vi "FPGA.vi"(8 "Servo PWM":i16, 9 "Motor PWM":i16=97, 13 "Slave Address":u8 format="%x", 15 "Data to send":u8[](array[numeric])=[0, 0] format="%b", 17 "Number of bytes":i16) -> (12 "Block Count":i16, 14 "Time of Flight Right":u32, 19 "Data bit array":bool[](array[boolean]), 20 "Time of Flight Front":u32, 24 "Time of Flight Back":u32, 26 "Time of Flight Left":u32)   [LabVIEW 2015]
uses:
  <vilib>/rvi/Emulation/niFpgaGetClockAttributes.vi
  <vilib>/rvi/Emulation/niFpgaSctlEmulationGetInTimedLoop.vi
  <vilib>/rvi/Emulation/niFpgaEmulationReportErrorSimple.vi
  <vilib>/rvi/eio/common/nirviEmuTemplateMethod_errors.vi
  <vilib>/rvi/Emulation/niFpgaCriticalErrorInLSC.vi
  <vilib>/rvi/Emulation/niFpgaProcessEmulError.vi
  <vilib>/eio/EIONode/EIONode.xnode
panel:
  out "Waveform Chart 2":i16(graph)
  out "Waveform Chart":i16(graph)
  in  "Read":bool=TRUE
  out "x*y 4":i16
  out "x*y 3":i16
  out "x*y 2":i16
  out "x*y":i16
  in  "stop":bool
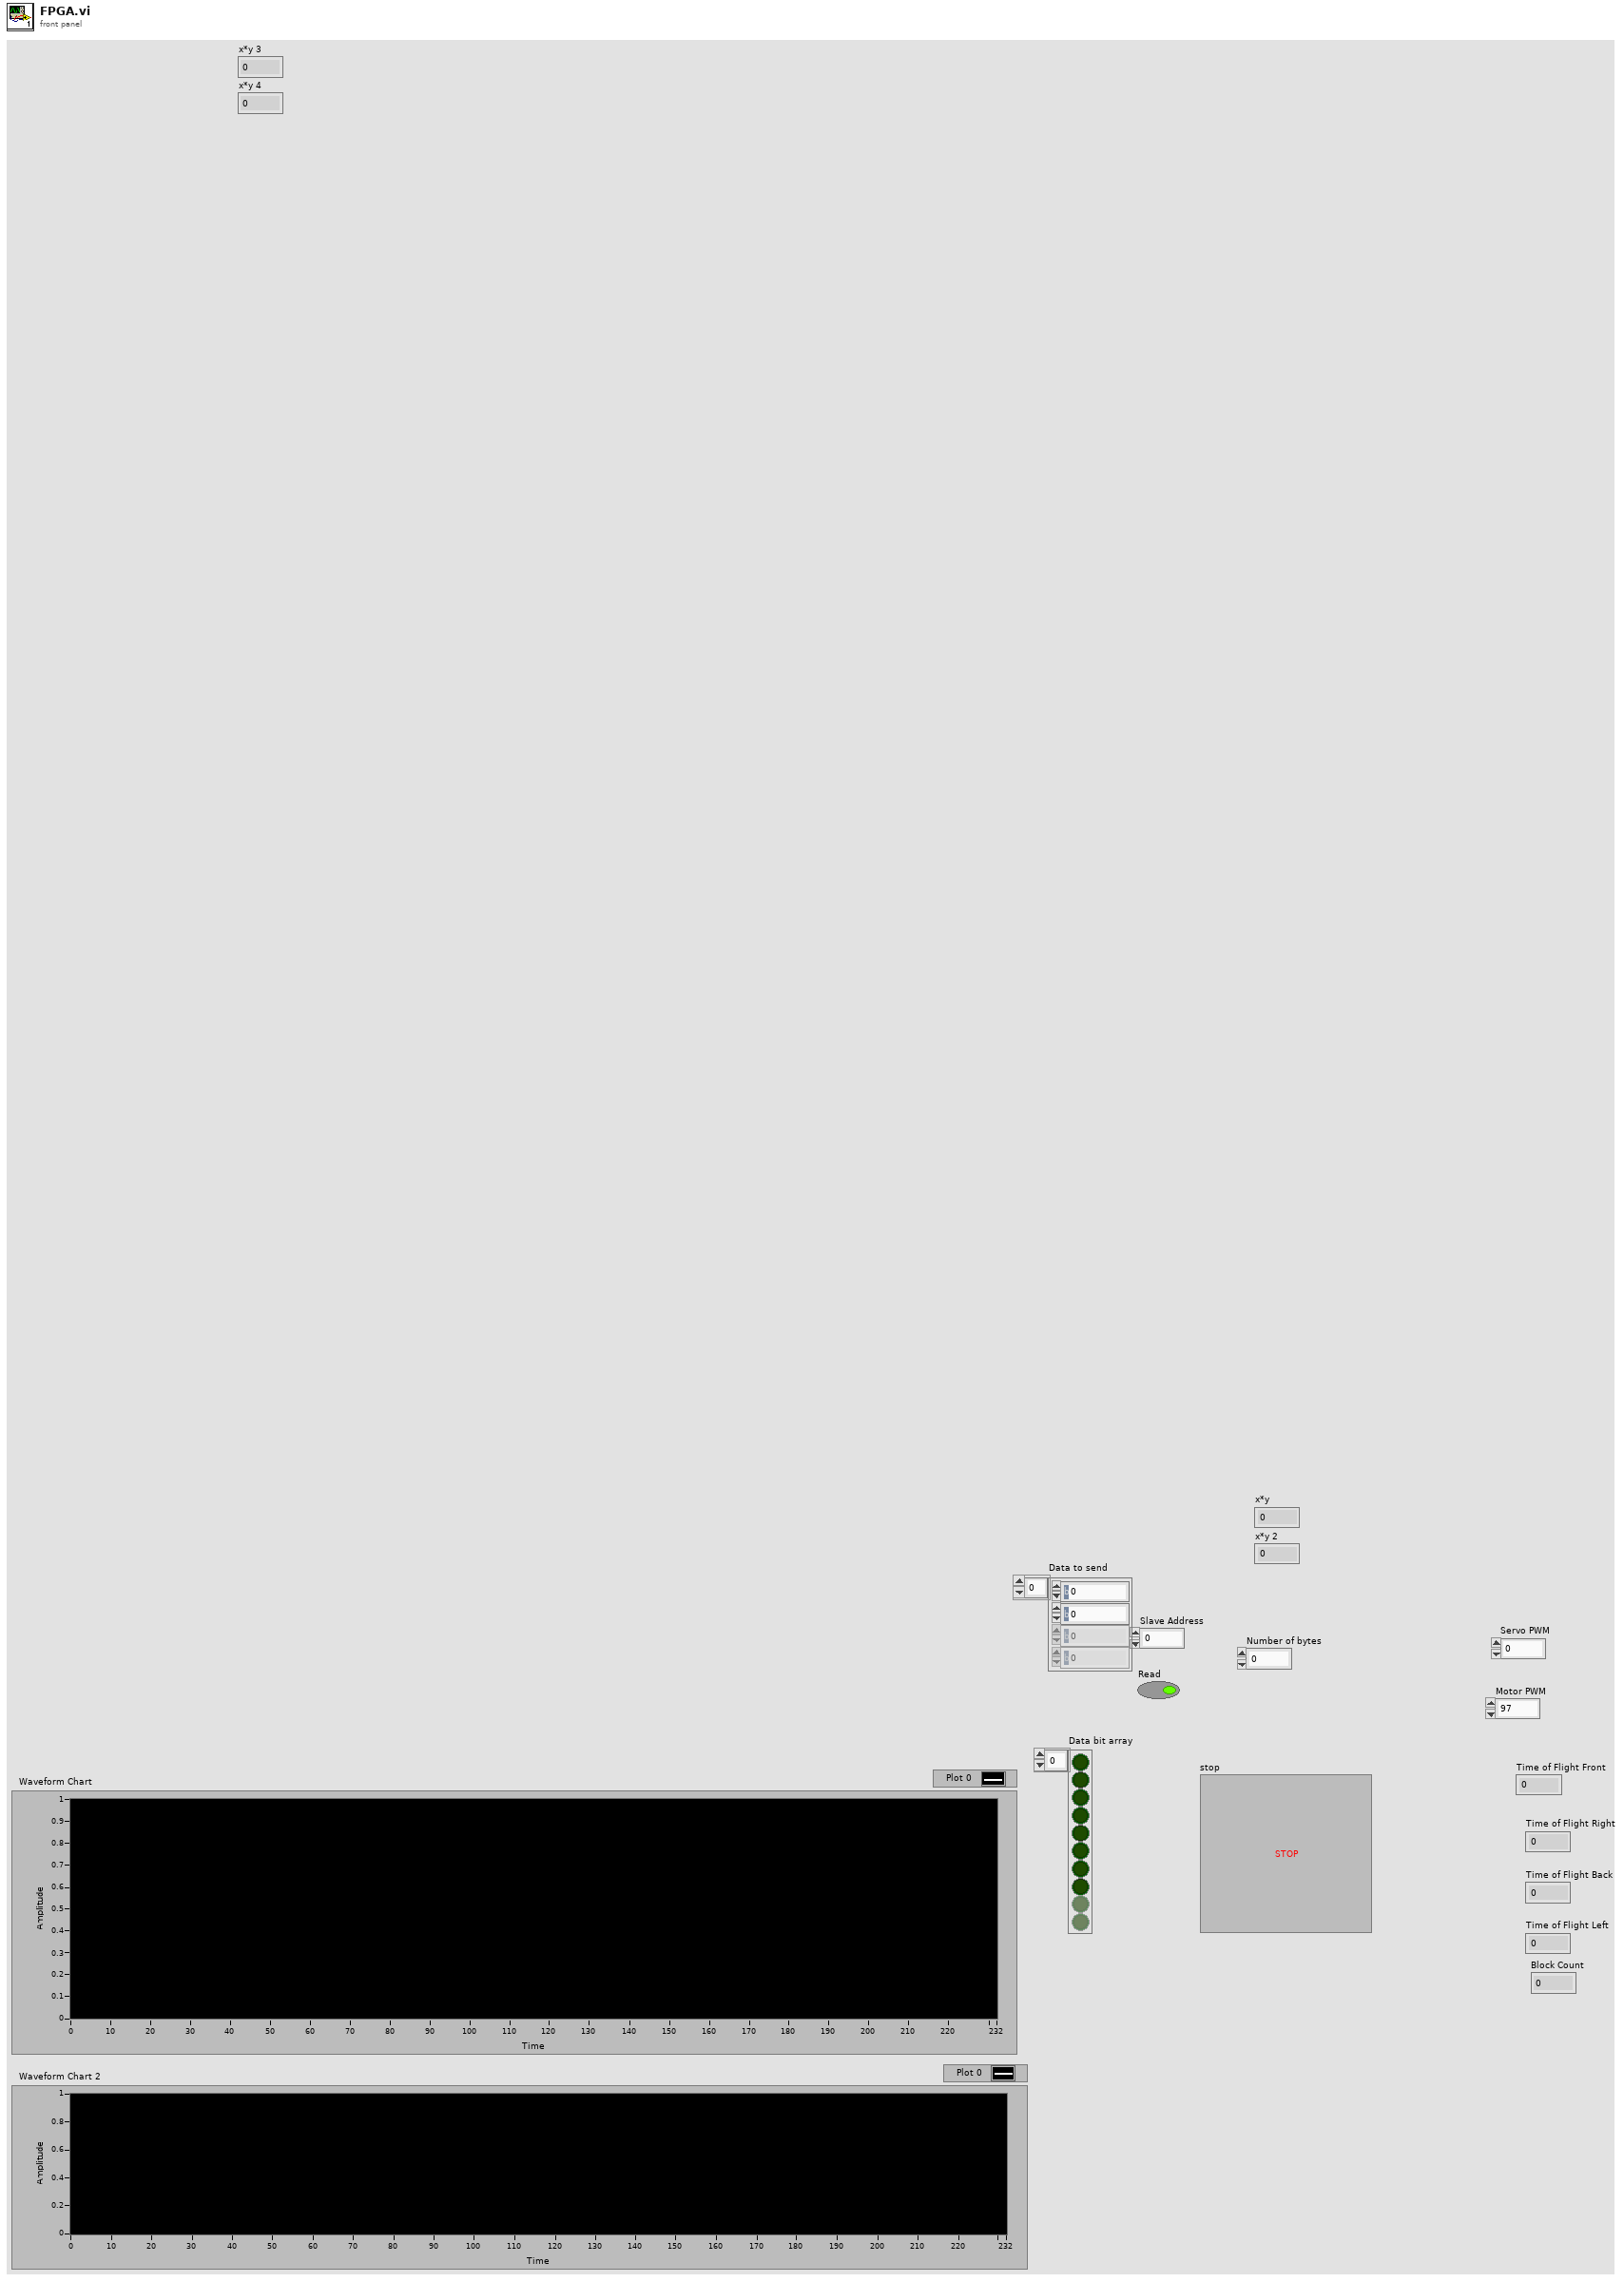
[diagram p1: front panel]
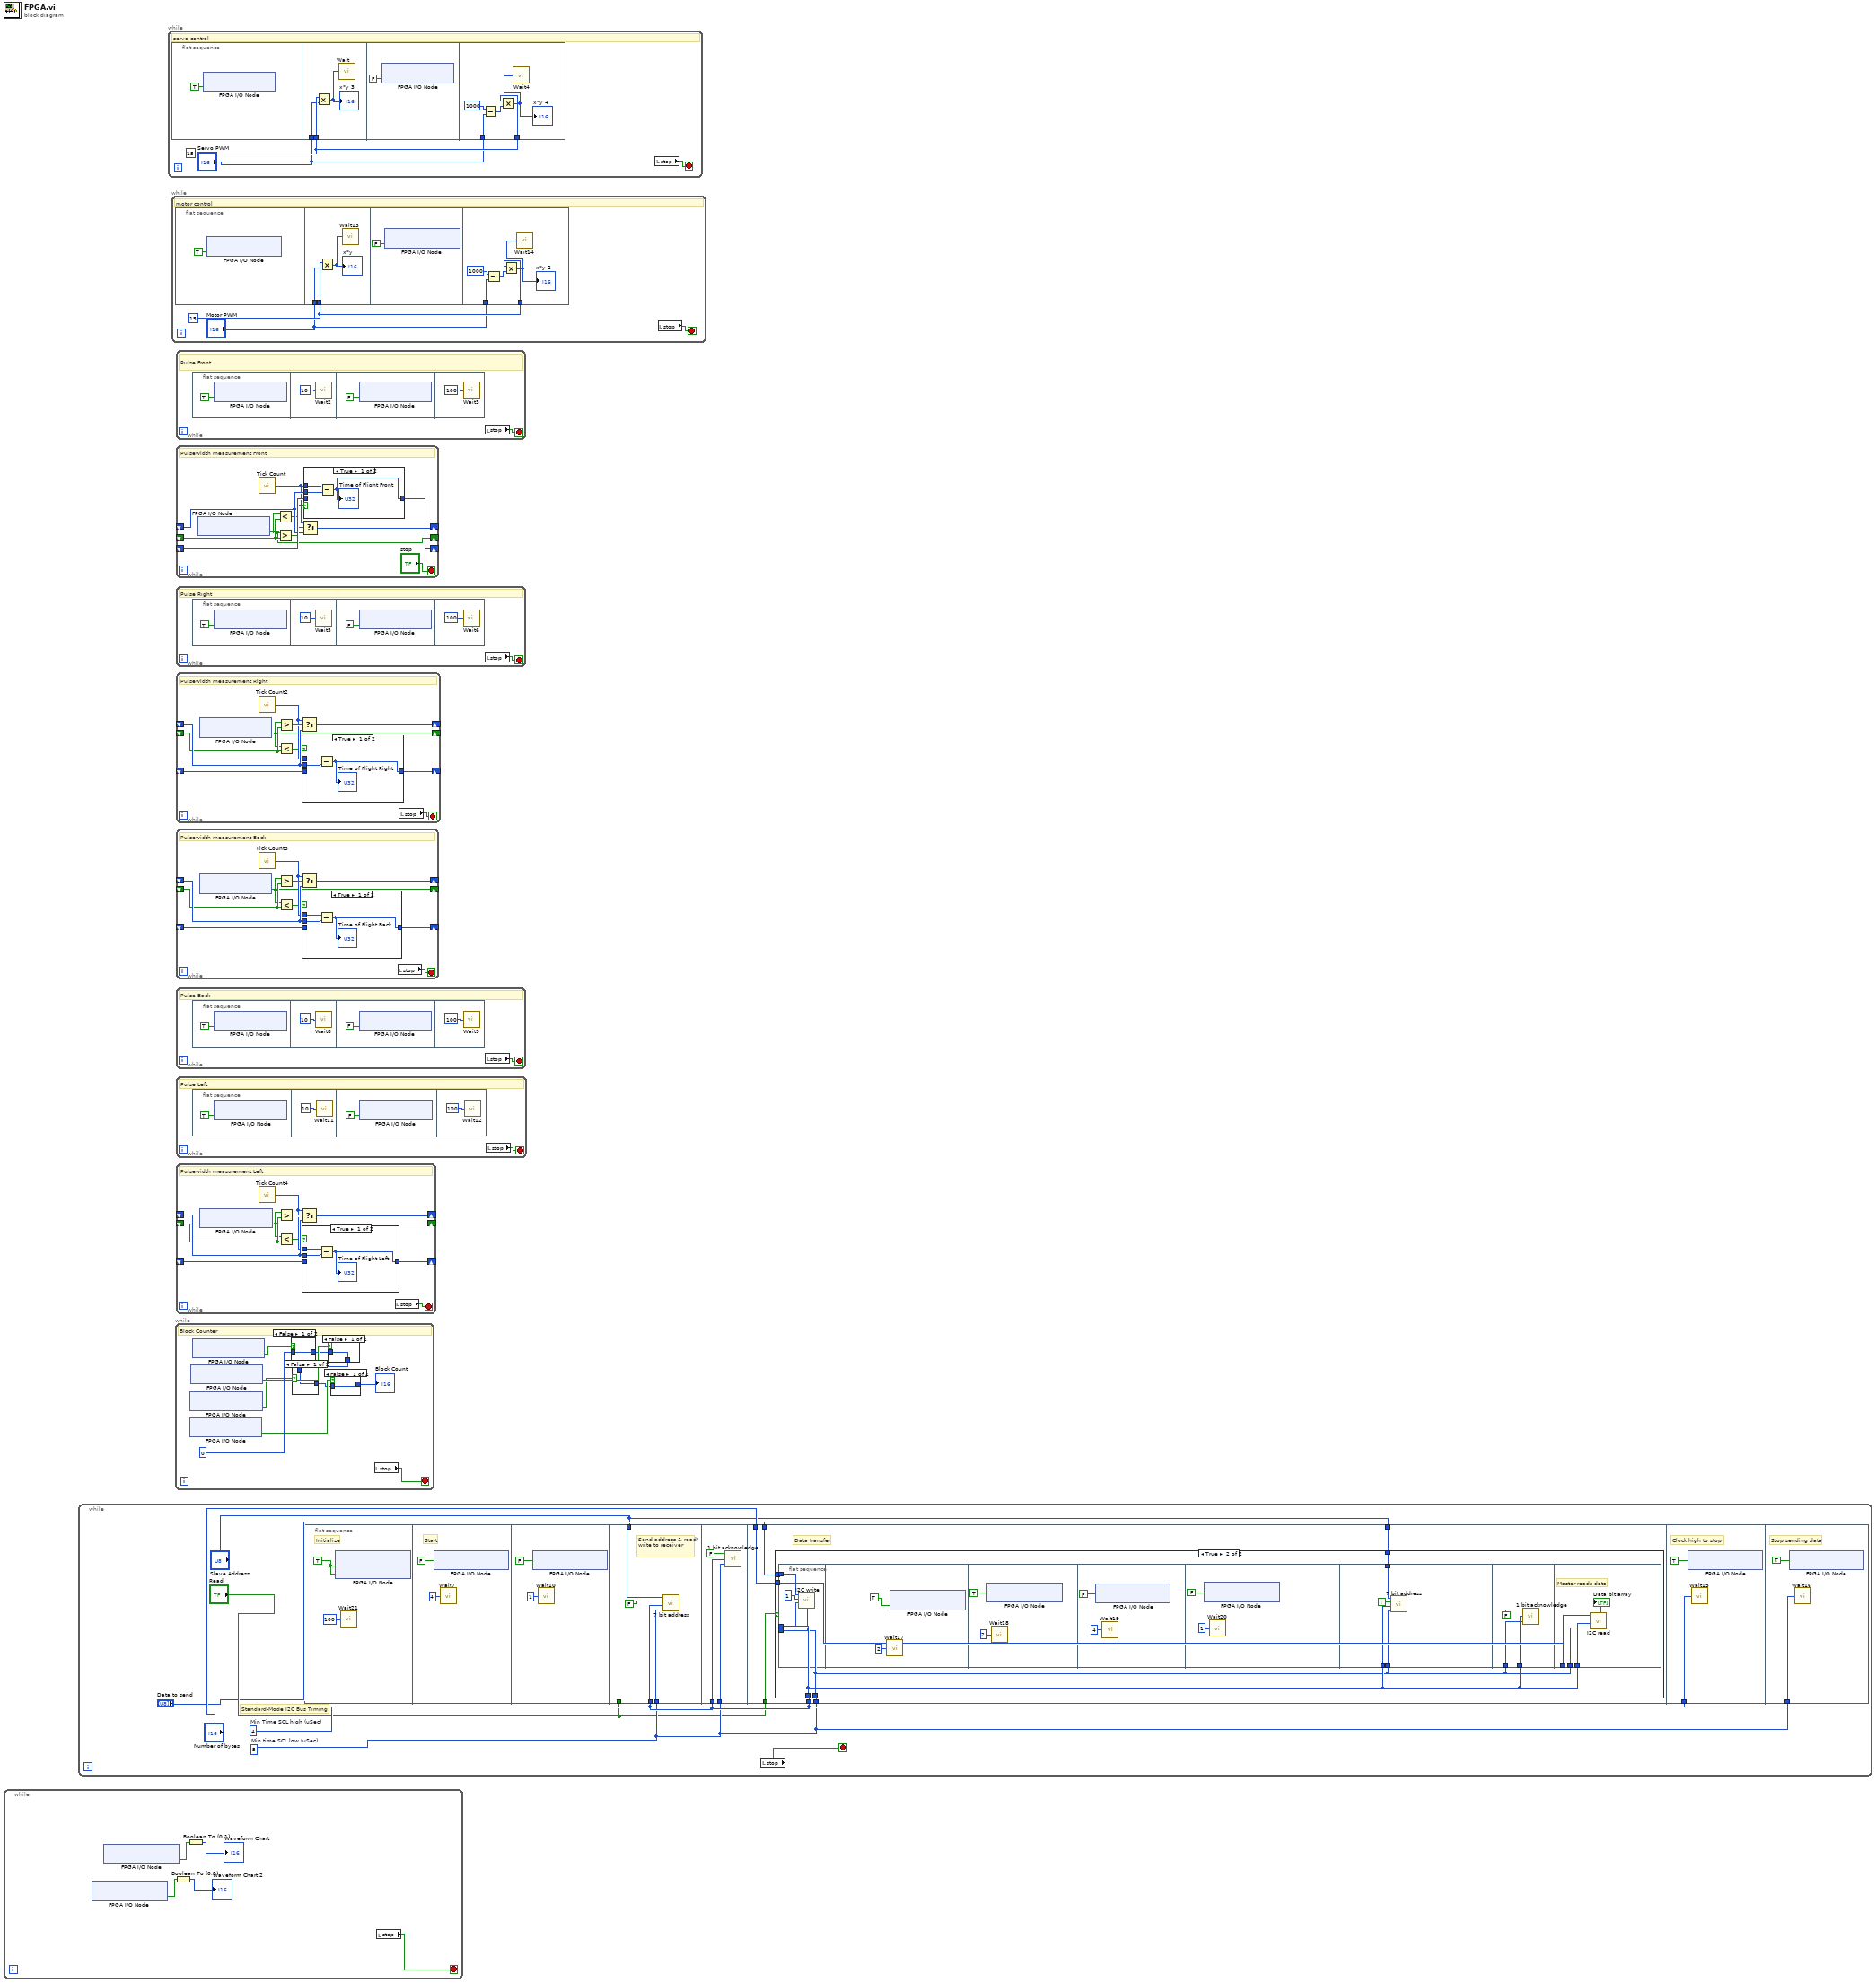
[diagram p0: block diagram]
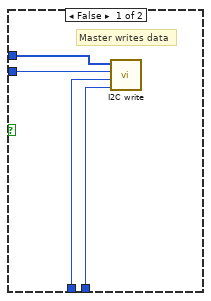
[diagram p2: hidden frame]
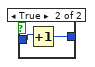
[diagram p3: hidden frame]
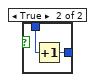
[diagram p4: hidden frame]
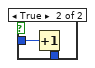
[diagram p5: hidden frame]
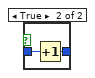
[diagram p6: hidden frame]
diagram:
  n1 = while {
    stop <- w5 stop-if-true
    n2 = xnode "FPGA I/O Node"() -> ("ConnectorB/DIO14"=w2:bool)  [unwired: 1 in, 1 out]
    n3 = xnode "FPGA I/O Node"() -> ("ConnectorB/DIO15"=w4:bool)  [unwired: 1 in, 1 out]
    n4 = Boolean To (0,1)(Boolean=w2) -> (0, 1=→"Waveform Chart 2":i16)
    n5 = Boolean To (0,1)(Boolean=w4) -> (0, 1=→"Waveform Chart":i16)
    n6 = local read "stop"() -> (w5:bool)
  }
  n7 = while {
    stop <- w12 stop-if-true
    w11 = 4  # Min Time SCL high (uSec)
    w10 = 5  # Min time SCL low (uSec)
    # "Standard-Mode I2C Bus Timing"
    n8 = flat-sequence {
      tunnel: "Read" -> [_]
      tunnel: w11 -> [w22]
      tunnel: w10 -> [w21]
      tunnel: "Slave Address" -> [w20]
      tunnel: w11 -> [w24]
      tunnel: w10 -> [w23]
      tunnel: "Read" -> [w31]
      tunnel: w11 -> [w30]
      tunnel: w10 -> [w29]
      tunnel: "Data to send" -> [w28]
      tunnel: "Number of bytes" -> [w27]
      tunnel: "Slave Address" -> [w26]
      tunnel: w11 -> [w64]
      tunnel: w10 -> [w67]
      frame #0 {
        w14 = TRUE ("Digital Out")
        # "Initialize"
        n9 = xnode "FPGA I/O Node"("ConnectorB/DIO15"=w14, "ConnectorB/DIO14"=w14) -> ()  [unwired: 2 in, 2 out]
        n10 = call "Wait21"("Count(uSec)"=u32 100) -> ()  [unwired: 1 out]
      }
      frame #1 {
        # "Start"
        n11 = xnode "FPGA I/O Node"("ConnectorB/DIO15"=FALSE ("Start Sending")) -> ()  [unwired: 1 in, 1 out]
        n12 = call "Wait7"("Count(uSec)"=u32 4) -> ()  [unwired: 1 out]
      }
      frame #2 {
        n13 = xnode "FPGA I/O Node"("ConnectorB/DIO14"=FALSE ("Digital Out")) -> ()  [unwired: 1 in, 1 out]
        n14 = call "Wait10"("Count(uSec)"=u32 1) -> ()  [unwired: 1 out]
      }
      frame #3 {
        # "Send address & read/write to receiver"
        n15 = call "7 bit address.vi"("Min time SCL low (uSec)"=w21, "Min Time SCL high (uSec)"=w22, "Read/Write?"=FALSE, "Receiver Address"=w20) -> ()
      }
      frame #4 {
        n16 = call "1 bit acknowledge.vi"("Min time SCL low (uSec)"=w23, "Min Time SCL high (uSec)"=w24, "Acknowledgement"=FALSE) -> ()
      }
      frame #5 {
        # "Data transfer"
        n17 = case shown="True" w31 {
          tunnel: w28 -> [w35 w40]
          tunnel: w27 -> [w34 w39]
          tunnel: w30 -> [w33 w37]
          tunnel: w29 -> [w32 w36]
          tunnel: w26 -> [_ w38]
          frame False {
            # "Master writes data"
            n18 = call "I2C write.vi"("Min time SCL low (uSec)"=w32, "Min Time SCL high (uSec)"=w33, "Number of Bytes"=w34, "Data to send"=w35) -> ()
          }
          frame True {
            n19 = flat-sequence {
              tunnel: w40 -> [w44]
              tunnel: w37 -> [w42]
              tunnel: w36 -> [w41]
              tunnel: w38 -> [w55]
              tunnel: w36 -> [w54]
              tunnel: w37 -> [w53]
              tunnel: w37 -> [w58]
              tunnel: w36 -> [w57]
              tunnel: w39 -> [w62]
              tunnel: w37 -> [w61]
              tunnel: w36 -> [w60]
              frame #0 {
                n20 = call "I2C write.vi"("Min time SCL low (uSec)"=w41, "Min Time SCL high (uSec)"=w42, "Number of Bytes"=i16 1, "Data to send"=w44) -> ()
              }
              frame #1 {
                n21 = call "Wait17"("Count(uSec)"=u32 2) -> ()  [unwired: 1 out]
                n22 = xnode "FPGA I/O Node"("ConnectorB/DIO15"=TRUE) -> ()  [unwired: 1 in, 1 out]
              }
              frame #2 {
                n23 = xnode "FPGA I/O Node"("ConnectorB/DIO14"=TRUE ("Digital Out")) -> ()  [unwired: 1 in, 1 out]
                n24 = call "Wait18"("Count(uSec)"=u32 2) -> ()  [unwired: 1 out]
              }
              frame #3 {
                n25 = xnode "FPGA I/O Node"("ConnectorB/DIO15"=FALSE ("Start Sending")) -> ()  [unwired: 1 in, 1 out]
                n26 = call "Wait19"("Count(uSec)"=u32 4) -> ()  [unwired: 1 out]
              }
              frame #4 {
                n27 = xnode "FPGA I/O Node"("ConnectorB/DIO14"=FALSE ("Digital Out")) -> ()  [unwired: 1 in, 1 out]
                n28 = call "Wait20"("Count(uSec)"=u32 1) -> ()  [unwired: 1 out]
              }
              frame #5 {
                n29 = call "7 bit address.vi"("Min time SCL low (uSec)"=w54, "Min Time SCL high (uSec)"=w53, "Read/Write?"=TRUE, "Receiver Address"=w55) -> ()
              }
              frame #6 {
                n30 = call "1 bit acknowledge.vi"("Min time SCL low (uSec)"=w57, "Min Time SCL high (uSec)"=w58, "Acknowledgement"=FALSE) -> ()
              }
              frame #7 {
                # "Master reads data"
                n31 = call "I2C read.vi"("Min time SCL low (uSec)"=w60, "Min Time SCL high (uSec)"=w61, "Number of Bytes"=w62) -> ("Data bit array"=→"Data bit array":bool[])
              }
            }
          }
        }
      }
      frame #6 {
        # "Clock high to stop"
        n32 = xnode "FPGA I/O Node"("ConnectorB/DIO14"=TRUE ("Digital Out")) -> ()  [unwired: 1 in, 1 out]
        n33 = call "Wait15"("Count(uSec)"=w64) -> ()  [unwired: 1 out]
      }
      frame #7 {
        # "Stop sending data"
        n34 = xnode "FPGA I/O Node"("ConnectorB/DIO15"=TRUE ("Digital Out")) -> ()  [unwired: 1 in, 1 out]
        n35 = call "Wait16"("Count(uSec)"=w67) -> ()  [unwired: 1 out]
      }
    }
    n36 = local read "stop"() -> (w12:bool)
  }
  n37 = while {
    stop <- w70 stop-if-true
    w69 = i16 15
    # "servo control"
    n38 = flat-sequence {
      tunnel: w69 -> [w74]
      tunnel: "Servo PWM" -> [w72]
      tunnel: w69 -> [w80]
      tunnel: "Servo PWM" -> [w78]
      frame #0 {
        n39 = xnode "FPGA I/O Node"("ConnectorB/DIO9"=TRUE ("ConnectorB/DIO10")) -> ()  [unwired: 1 in, 1 out]
      }
      frame #1 {
        n40 = Multiply(x=w74, y=w72) -> (x*y=w73:i16)
        "x*y 3" <- w73
        n41 = call "Wait"("Count(uSec)"=w73) -> ()  [unwired: 1 out]
      }
      frame #2 {
        n42 = xnode "FPGA I/O Node"("ConnectorB/DIO9"=FALSE ("ConnectorB/DIO10")) -> ()  [unwired: 1 in, 1 out]
      }
      frame #3 {
        n43 = Subtract(x=i16 1000, y=w78) -> (x-y=w77:i16)
        n44 = Multiply(x=w80, y=w77) -> (x*y=w76:i16)
        "x*y 4" <- w76
        n45 = call "Wait4"("Count(uSec)"=w76) -> ()  [unwired: 1 out]
      }
    }
    n46 = local read "stop"() -> (w70:bool)
  }
  n47 = while {
    stop <- w83 stop-if-true
    w82 = i16 15
    # "motor control"
    n48 = flat-sequence {
      tunnel: w82 -> [w87]
      tunnel: "Motor PWM" -> [w85]
      tunnel: w82 -> [w93]
      tunnel: "Motor PWM" -> [w91]
      frame #0 {
        n49 = xnode "FPGA I/O Node"("ConnectorB/DIO10"=TRUE) -> ()  [unwired: 1 in, 1 out]
      }
      frame #1 {
        n50 = Multiply(x=w87, y=w85) -> (x*y=w86:i16)
        "x*y" <- w86
        n51 = call "Wait13"("Count(uSec)"=w86) -> ()  [unwired: 1 out]
      }
      frame #2 {
        n52 = xnode "FPGA I/O Node"("ConnectorB/DIO10"=FALSE) -> ()  [unwired: 1 in, 1 out]
      }
      frame #3 {
        n53 = Subtract(x=i16 1000, y=w91) -> (x-y=w90:i16)
        n54 = Multiply(x=w93, y=w90) -> (x*y=w89:i16)
        "x*y 2" <- w89
        n55 = call "Wait14"("Count(uSec)"=w89) -> ()  [unwired: 1 out]
      }
    }
    n56 = local read "stop"() -> (w83:bool)
  }
  n57 = while {
    stop <- w103 stop-if-true
    # "Block Counter"
    n58 = xnode "FPGA I/O Node"() -> ("ConnectorC/DIO2"=w96:bool)  [unwired: 1 in, 1 out]
    n59 = xnode "FPGA I/O Node"() -> ("ConnectorC/DIO4"=w98:bool)  [unwired: 1 in, 1 out]
    n60 = xnode "FPGA I/O Node"() -> ("ConnectorC/DIO5"=w100:bool)  [unwired: 1 in, 1 out]
    n61 = xnode "FPGA I/O Node"() -> ("ConnectorC/DIO6"=w102:bool)  [unwired: 1 in, 1 out]
    n62 = case shown="False" w102 {
      tunnel: i16 0 -> [w113 w115]
      tunnel: [w113 w114] -> w99
      frame False {
      }
      frame True {
        n63 = Increment(x=w115) -> (x+1=w114:i16)
      }
    }
    n64 = case shown="False" w100 {
      tunnel: w99 -> [w110 w112]
      tunnel: [w110 w111] -> w97
      frame False {
      }
      frame True {
        n65 = Increment(x=w112) -> (x+1=w111:i16)
      }
    }
    n66 = case shown="False" w98 {
      tunnel: w97 -> [w107 w109]
      tunnel: [w107 w108] -> w95
      frame False {
      }
      frame True {
        n67 = Increment(x=w109) -> (x+1=w108:i16)
      }
    }
    n68 = case shown="False" w96 {
      tunnel: w95 -> [w104 w106]
      tunnel: [w104 w105] -> w94
      frame False {
      }
      frame True {
        n69 = Increment(x=w106) -> (x+1=w105:i16)
      }
    }
    "Block Count" <- w94
    n70 = local read "stop"() -> (w103:bool)
  }
  n71 = while {
    stop <- w116 stop-if-true
    # "Pulse Front"
    n72 = flat-sequence {
      frame #0 {
        n73 = xnode "FPGA I/O Node"("ConnectorB/DIO4"=TRUE) -> ()  [unwired: 1 in, 1 out]
      }
      frame #1 {
        n74 = call "Wait2"("Count(uSec)"=u32 10 ("Count(mSec)")) -> ()  [unwired: 1 out]
      }
      frame #2 {
        n75 = xnode "FPGA I/O Node"("ConnectorB/DIO4"=FALSE) -> ()  [unwired: 1 in, 1 out]
      }
      frame #3 {
        n76 = call "Wait3"("Count(mSec)"=u32 100) -> ()  [unwired: 1 out]
      }
    }
    n77 = local read "stop"() -> (w116:bool)
  }
  n78 = while "Pulsewidth Measurement + Sound Output" {
    shift-left: _ -> [w130]
    shift-right: [w122] -> _
    shift-left: _ -> [w129]
    shift-right: [w128] -> _
    shift-left: _ -> [w126]
    shift-right: [w123] -> _
    stop <- "stop" stop-if-true
    # "Pulsewidth measurement Front"
    n79 = xnode "FPGA I/O Node"() -> ("ConnectorB/DIO7"=w123:bool)  [unwired: 1 in, 1 out]
    n80 = call "Tick Count"() -> ("Tick Count(uSec)"=w125:u32)
    n81 = Less?(x=w123, y=w126) -> (x < y?=w124:bool)
    n82 = Greater?(x=w123, y=w126) -> (0:w127:bool)
    n83 = Select(t=w125, s=w127, f=w129) -> (s? t:f=w128:u32)
    n84 = case shown="True" w124 {
      tunnel: w130 -> [_ w134]
      tunnel: w125 -> [w132 _]
      tunnel: w129 -> [w133 _]
      tunnel: [w131 w134] -> w122
      frame True {
        n85 = Subtract(x=w132, y=w133) -> (x-y=w131:u32)
        "Time of Flight Front" <- w131
      }
      frame False {
      }
    }
  }
  n86 = while {
    stop <- w135 stop-if-true
    # "Pulse Right"
    n87 = flat-sequence {
      frame #0 {
        n88 = xnode "FPGA I/O Node"("ConnectorB/DIO3"=TRUE ("ConnectorB/DIO4")) -> ()  [unwired: 1 in, 1 out]
      }
      frame #1 {
        n89 = call "Wait5"("Count(uSec)"=u32 10 ("Count(mSec)")) -> ()  [unwired: 1 out]
      }
      frame #2 {
        n90 = xnode "FPGA I/O Node"("ConnectorB/DIO3"=FALSE ("ConnectorB/DIO4")) -> ()  [unwired: 1 in, 1 out]
      }
      frame #3 {
        n91 = call "Wait6"("Count(mSec)"=u32 100) -> ()  [unwired: 1 out]
      }
    }
    n92 = local read "stop"() -> (w135:bool)
  }
  n93 = while "Pulsewidth Measurement + Sound Output" {
    shift-left: _ -> [w149]
    shift-right: [w144] -> _
    shift-left: _ -> [w148]
    shift-right: [w147] -> _
    shift-left: _ -> [w145]
    shift-right: [w141] -> _
    stop <- w140 stop-if-true
    # "Pulsewidth measurement Right"
    n94 = xnode "FPGA I/O Node"() -> ("ConnectorB/DIO0"=w141:bool)  [unwired: 1 in, 1 out]
    n95 = call "Tick Count2"() -> ("Tick Count(uSec)"=w143:u32)
    n96 = Greater?(x=w141, y=w145) -> (0:w146:bool)
    n97 = Less?(x=w141, y=w145) -> (x < y?=w142:bool)
    n98 = Select(t=w143, s=w146, f=w148) -> (s? t:f=w147:u32)
    n99 = case shown="True" w142 {
      tunnel: w149 -> [_ w153]
      tunnel: w143 -> [w151 _]
      tunnel: w148 -> [w152 _]
      tunnel: [w150 w153] -> w144
      frame True {
        n100 = Subtract(x=w151, y=w152) -> (x-y=w150:u32)
        "Time of Flight Right" <- w150
      }
      frame False {
      }
    }
    n101 = local read "stop"() -> (w140:bool)
  }
  n102 = while "Pulsewidth Measurement + Sound Output" {
    shift-left: _ -> [w163]
    shift-right: [w158] -> _
    shift-left: _ -> [w162]
    shift-right: [w161] -> _
    shift-left: _ -> [w159]
    shift-right: [w155] -> _
    stop <- w154 stop-if-true
    # "Pulsewidth measurement Back"
    n103 = xnode "FPGA I/O Node"() -> ("ConnectorB/DIO1"=w155:bool)  [unwired: 1 in, 1 out]
    n104 = call "Tick Count3"() -> ("Tick Count(uSec)"=w157:u32)
    n105 = Greater?(x=w155, y=w159) -> (0:w160:bool)
    n106 = Less?(x=w155, y=w159) -> (x < y?=w156:bool)
    n107 = Select(t=w157, s=w160, f=w162) -> (s? t:f=w161:u32)
    n108 = case shown="True" w156 {
      tunnel: w163 -> [_ w167]
      tunnel: w157 -> [w165 _]
      tunnel: w162 -> [w166 _]
      tunnel: [w164 w167] -> w158
      frame True {
        n109 = Subtract(x=w165, y=w166) -> (x-y=w164:u32)
        "Time of Flight Back" <- w164
      }
      frame False {
      }
    }
    n110 = local read "stop"() -> (w154:bool)
  }
  n111 = while {
    stop <- w168 stop-if-true
    # "Pulse Back"
    n112 = flat-sequence {
      frame #0 {
        n113 = xnode "FPGA I/O Node"("ConnectorB/DIO2"=TRUE ("ConnectorB/DIO4")) -> ()  [unwired: 1 in, 1 out]
      }
      frame #1 {
        n114 = call "Wait8"("Count(uSec)"=u32 10 ("Count(mSec)")) -> ()  [unwired: 1 out]
      }
      frame #2 {
        n115 = xnode "FPGA I/O Node"("ConnectorB/DIO2"=FALSE ("ConnectorB/DIO4")) -> ()  [unwired: 1 in, 1 out]
      }
      frame #3 {
        n116 = call "Wait9"("Count(mSec)"=u32 100) -> ()  [unwired: 1 out]
      }
    }
    n117 = local read "stop"() -> (w168:bool)
  }
  n118 = while {
    stop <- w173 stop-if-true
    # "Pulse Left"
    n119 = flat-sequence {
      frame #0 {
        n120 = xnode "FPGA I/O Node"("ConnectorC/DIO1"=TRUE ("ConnectorB/DIO4")) -> ()  [unwired: 1 in, 1 out]
      }
      frame #1 {
        n121 = call "Wait11"("Count(uSec)"=u32 10 ("Count(mSec)")) -> ()  [unwired: 1 out]
      }
      frame #2 {
        n122 = xnode "FPGA I/O Node"("ConnectorC/DIO1"=FALSE ("ConnectorB/DIO4")) -> ()  [unwired: 1 in, 1 out]
      }
      frame #3 {
        n123 = call "Wait12"("Count(mSec)"=u32 100) -> ()  [unwired: 1 out]
      }
    }
    n124 = local read "stop"() -> (w173:bool)
  }
  n125 = while "Pulsewidth Measurement + Sound Output" {
    shift-left: _ -> [w187]
    shift-right: [w179] -> _
    shift-left: _ -> [w186]
    shift-right: [w185] -> _
    shift-left: _ -> [w183]
    shift-right: [w180] -> _
    stop <- w178 stop-if-true
    # "Pulsewidth measurement Left"
    n126 = xnode "FPGA I/O Node"() -> ("ConnectorC/DIO0"=w180:bool)  [unwired: 1 in, 1 out]
    n127 = call "Tick Count4"() -> ("Tick Count(uSec)"=w182:u32)
    n128 = Greater?(x=w180, y=w183) -> (0:w184:bool)
    n129 = Less?(x=w180, y=w183) -> (x < y?=w181:bool)
    n130 = Select(t=w182, s=w184, f=w186) -> (s? t:f=w185:u32)
    n131 = case shown="True" w181 {
      tunnel: w187 -> [_ w191]
      tunnel: w182 -> [w189 _]
      tunnel: w186 -> [w190 _]
      tunnel: [w188 w191] -> w179
      frame True {
        n132 = Subtract(x=w189, y=w190) -> (x-y=w188:u32)
        "Time of Flight Left" <- w188
      }
      frame False {
      }
    }
    n133 = local read "stop"() -> (w178:bool)
  }
